vi "parse handshake message.vi"(8 "error in":errorcluster, 11 "String":string) -> (0 "error out":errorcluster, 1 "headers":map{string, string[]}(c390), 2 "HTTP method":T1, 3 "URL":string, 4 "HTTP protocol version":T2)   [LabVIEW 2019, in "WebSocket Server Toolkit.lvlib"]
uses:
  WebSocket Server Toolkit.lvlib
  types/HTTP Protocol Version.ctl
  types/HTTP Request Method.ctl
  <vilib>/AdvancedString/Delimited String to 1D String Array.vi
  <vilib>/Utility/error.llb/Trim Whitespace.vi
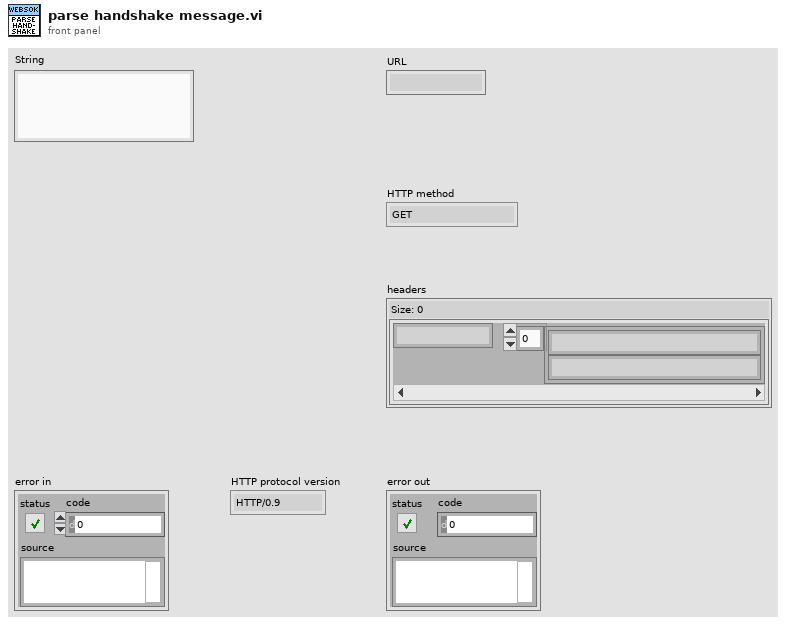
[diagram p1: front panel]
types:
  T1 = typedef "WebSocket Server Toolkit.lvlib/HTTP Request Method.ctl" = enum16{"GET", "HEAD", "POST", "PUT", "DELETE", "CONNECT", "OPTIONS", "TRACE", "PATCH"}
  T2 = typedef "WebSocket Server Toolkit.lvlib/HTTP Protocol Version.ctl" = enum16{"HTTP/0.9", "HTTP/1.0", "HTTP/1.1", "HTTP/2.0", "HTTP/3.0"}
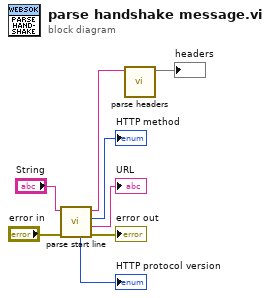
[diagram p0: block diagram]
diagram:
  n1 = call "parse start line.vi"("error in"="error in", "String"="String") -> ("error out"=→"error out":errorcluster, "URL"=→"URL":string, "HTTP method"=→"HTTP method":T1, "remaining string"=w7:string, "HTTP protocol version"=→"HTTP protocol version":T2)  [unwired: 4 in, 1 out]
  n2 = call "parse headers.vi"("String"=w7) -> ("headers"=→"headers":map{string, string[]})  [unwired: 10 in]
